vi "Dashboard Main.vi"() -> ()   [LabVIEW 2020]
uses:
  <vilib>/event_ctls.llb/eventvkey.ctl
  52f2dcef-b32f-41dc-9262-467f65fbdc6c.vi
  68ab9017-3ada-4b2c-b8c3-c0fcfab6ce46.vi
  <vilib>/Rock Robotics/Network Tables/NT Write Boolean.vi
  <vilib>/Rock Robotics/WPI/Dashboard/WPI_DashboardLogging Global.vi
  <vilib>/Analysis/NI_AALBase.lvlib
  <vilib>/Rock Robotics/Network Tables/NT Write Numeric Array.vi
panel:
  out "NT Connection":bool
  in  "Camera Settings Right":T1={"Frame Rate"=30, "Compression"=30, "Size"=1, "DB Camera Config"=FALSE} {"Frame Rate" scale=1.0..30.0; "Compression" scale=100.0..-1.0; "Size" items=["640x480", "320x240", "160x120"]}
  in  "Camera Name Right":string(combo)="No Camera Selection"
  out "Camera Perf":string
  in  "TCP":refnum<k5>
  in  "Rec Mode":enum32{"Stop", "Record", "Playback"}(radio)
  out "Robot IP":string
  out "Image Message":string="Timeout in Camera Communications"
  in  "Dashboard Tab":T2(tab)
  in  "Reset Climb":bool
  in  "Robot Selector":u16(ring) items=["2468", "2687"]
  out "Climb State":u16(ring) items=["Flip Hooks", "Rest Bar", "Tilt Back", "Tilt to Bar", "Grab Bar", "Pull Up"]
  out "Current Bar":u16(ring) items=["Ground", "Mid", "High", "Traverse"]
  in  "Calibrate (Reset Pods)":bool
  in  "Manual Paths":string[](array[string])
  in  "Ramping On?":bool
  in  "Max Rotation":dbl=540.0
  in  "Max Translation":dbl=15.0
  in  "Deadband":dbl=0.02
  out "Top Flywheel Voltage":dbl
  out "Auto Picture":picture
  in  "Auto Calibrate On?":bool=TRUE
  in  "Reset Hood":bool
  out "Main Flywheel RPM":dbl
  out "Hood Position":dbl
  in  "Auto Selector":T3(ring)
  out "IMU":dbl(knob) scale=-180.0..180.0
  out "Pivot Position":dbl
  out "Extension Position":dbl
  in  "Select Auto":string(combo)="Select Autonomous ..."
  out "Mode":T4(ring)=enum."Auto Disabled"
  out "Right Camera Perf":cluster{"Bandwidth (Mbps)":dbl, "FPS":dbl}
  in  "CheckList":i32(listbox)
  out "Climb State":u16(ring) items=["Flip Hooks", "Rest Bar", "Tilt Back", "Tilt to Bar", "Grab Bar", "Pull Up"]
  out "Current Shot":u16(ring) items=["Off", "Tarmac/Wall", "Protected"]
  out "Field Centric On?":bool
  out "Auto Align?":bool
  out "Background 2":bool
  out "Camera Image Right":T5(plugin-control)
  out "Tree":string(tree)
  out "Background":bool
  # "HW"
  # "IMU"
  # "Climb"
  # "Setup"
  # "Swerve"
  # "Shooter"
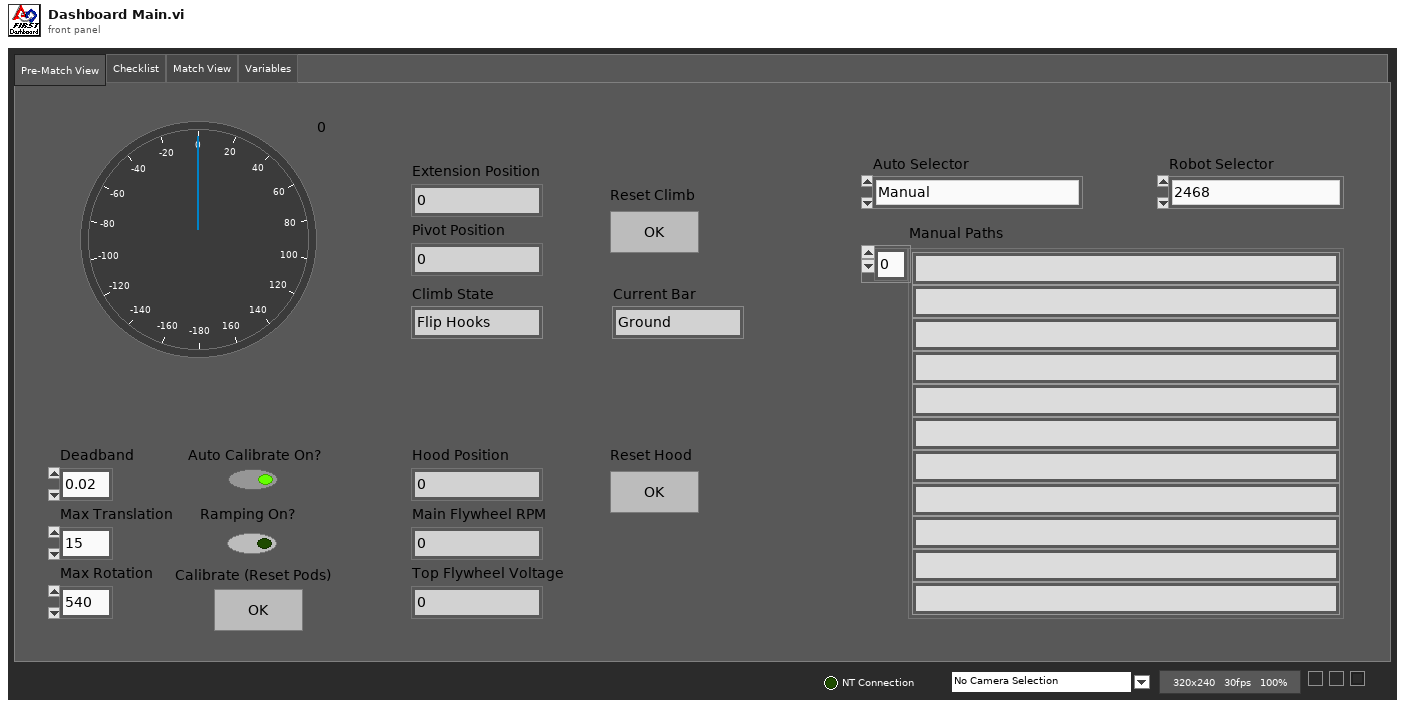
[diagram p1: front panel]
types:
  T1 = cluster{"Frame Rate":i32, "Compression":i32, "Size":u16, "DB Camera Config":bool}
  T2 = enum32{"Pre-Match View", "Checklist", "Match View", "Variables"}
  T3 = enum16{"Manual", "2 Ball Right", "5 Ball", "4 Ball Left", "4 Ball Right", "3 Ball", "2 Ball Left", "1 Ball"}
  T4 = enum8{"Tele-Op Disabled", "Tele-Op Enabled", "Auto Disabled", "Auto Enabled", "Test Disabled", "Test Enabled", "Disconnected", "No Code", "E-Stop"}
  T5 = typedef "IMAQ Image.ctl" = refnum<image>
  T6 = cluster{"Save Path":path, "Interval (s)":dbl, "Keep":i32}
  T7 = typedef "Image Type" = u32
  T8 = cluster{"IDs":cluster{"RPC field ID":u16, "Unique ID":u16}, "String":string}
  T9 = cluster{"Dashboard Tab":refnum<vi>, "Background":refnum<vi>, "Rec Mode":refnum<vi>, "Tree":refnum<vi>, "Camera Perf":refnum<vi>, "Camera Settings Right":refnum<vi>, "Camera Name Right":refnum<vi>, "Camera Image Right":refnum<vi>}
  T10 = cluster{"Global Rectangle":i32[], "Contours":cluster{"Contour Type":u32, "ROI Type":u32, "Points":i32[]}[]}
  T11 = cluster{"Camera Name Right":string, string, "Saved DB Images Info":cluster{"Save Path":path, "Interval (s)":dbl, "Keep":i32}}
  T12 = cluster{"Error Strings":string, "Disable Counts":cluster{u16, u16}, "Rail Faults":cluster{u16, u16, u16}, "Robot IP":string, "DB Mode":u8, "Event Info":cluster{"Name":string, "Type":u8, "Number":u16, "Replay":u8}}
  T13 = cluster{"Storage":cluster{"Disk Free":u64, "RAM Block":u32, "RAM free":u32}, "CPU Utilization":cluster{"CPU % ISR":sgl, "CPU % Time Crit":sgl, "CPU % Timed Str":sgl, "CPU % High":sgl, "CPU % Above":sgl, "CPU % Normal":sgl, "CPU % Low":sgl}, "CAN":cluster{"% Bus Utilization":sgl, "Bus Off Cnt":u32, "TX_FIFO Full Cnt":u32, "Receive Error Cnt":u8, "Transmit Error Cnt":u8}, "HID":cluster{"HID Outputs":u32, "Rumble Low":u16, "Rumble High":u16}[]}
  T14 = cluster{"Status bits":cluster{"Test Mode":bool, "Autonomous":bool, "Enabled":bool, "Code Start":bool, "Brownout":bool, "Reserved 2":bool, "Reserved 3":bool, "E-Stop":bool}, "Code Trace":cluster{"Disabled":bool, "TeleOp":bool, "Auto":bool, "Test":bool}, "Controller Type":enum16{"unknown", "cRIO", "roboRio"}, "Code?":enum16{"unknown", "noCode", "code"}, "Battery V":dbl}
  T15 = cluster{"Control Bits":cluster{"TestMode":bool, "Autonomous":bool, "Enabled":bool, "FMS Present":bool, bool, bool, bool, "E-Stop":bool}, "Team Station ":u8, "Countdown":sgl, "Joystick Values":cluster{"Axes":dbl[], "Buttons":bool[], "POVs":i16[]}[]}
  T16 = typedef "imagedata.ctl" = cluster{"image type":i32, "image depth":i32, "image":u8[], "mask":u8[], "colors":u32[], "Rectangle":cluster{"left":i16, "top":i16, "right":i16, "bottom":i16}}
  T17 = cluster{"Operation":enum16{"Update", "Clear"}, "Color Box":u32}[]
  T18 = typedef "eventvkey.ctl" = enum16{"ASCII", "Enter", "Return", "Shift", "Ctrl", "Alt", "Cmd", "Opt", "Caps", "NumLock", "Clear", "Break", "Up", "Down", "Left", "Right", "Insert", "Delete", "Home", "End", "PageUp", "PageDown", "Escape", "Help", "Pause", "ScrollLock", "F1", "F2", "F3", "F4", "F5", "F6", "F7", "F8", "F9", "F10", "F11", "F12", "F13", "F14", "F15", "F16", "F17", "F18", "F19", "F20", "F21", "F22", "F23", "F24", "Play", "VolumeUp", "VolumeDown", "Mute", "Two Byte Char"}
  T19 = cluster{"Image Size":bool, "Image Type":bool, "Pixel Value":bool, "ROI Information":bool, "Zoom Factor":bool}
  T20 = cluster{"Shift":bool, "Ctrl":bool, "Alt":bool, "Cmd":bool, "Opt":bool}
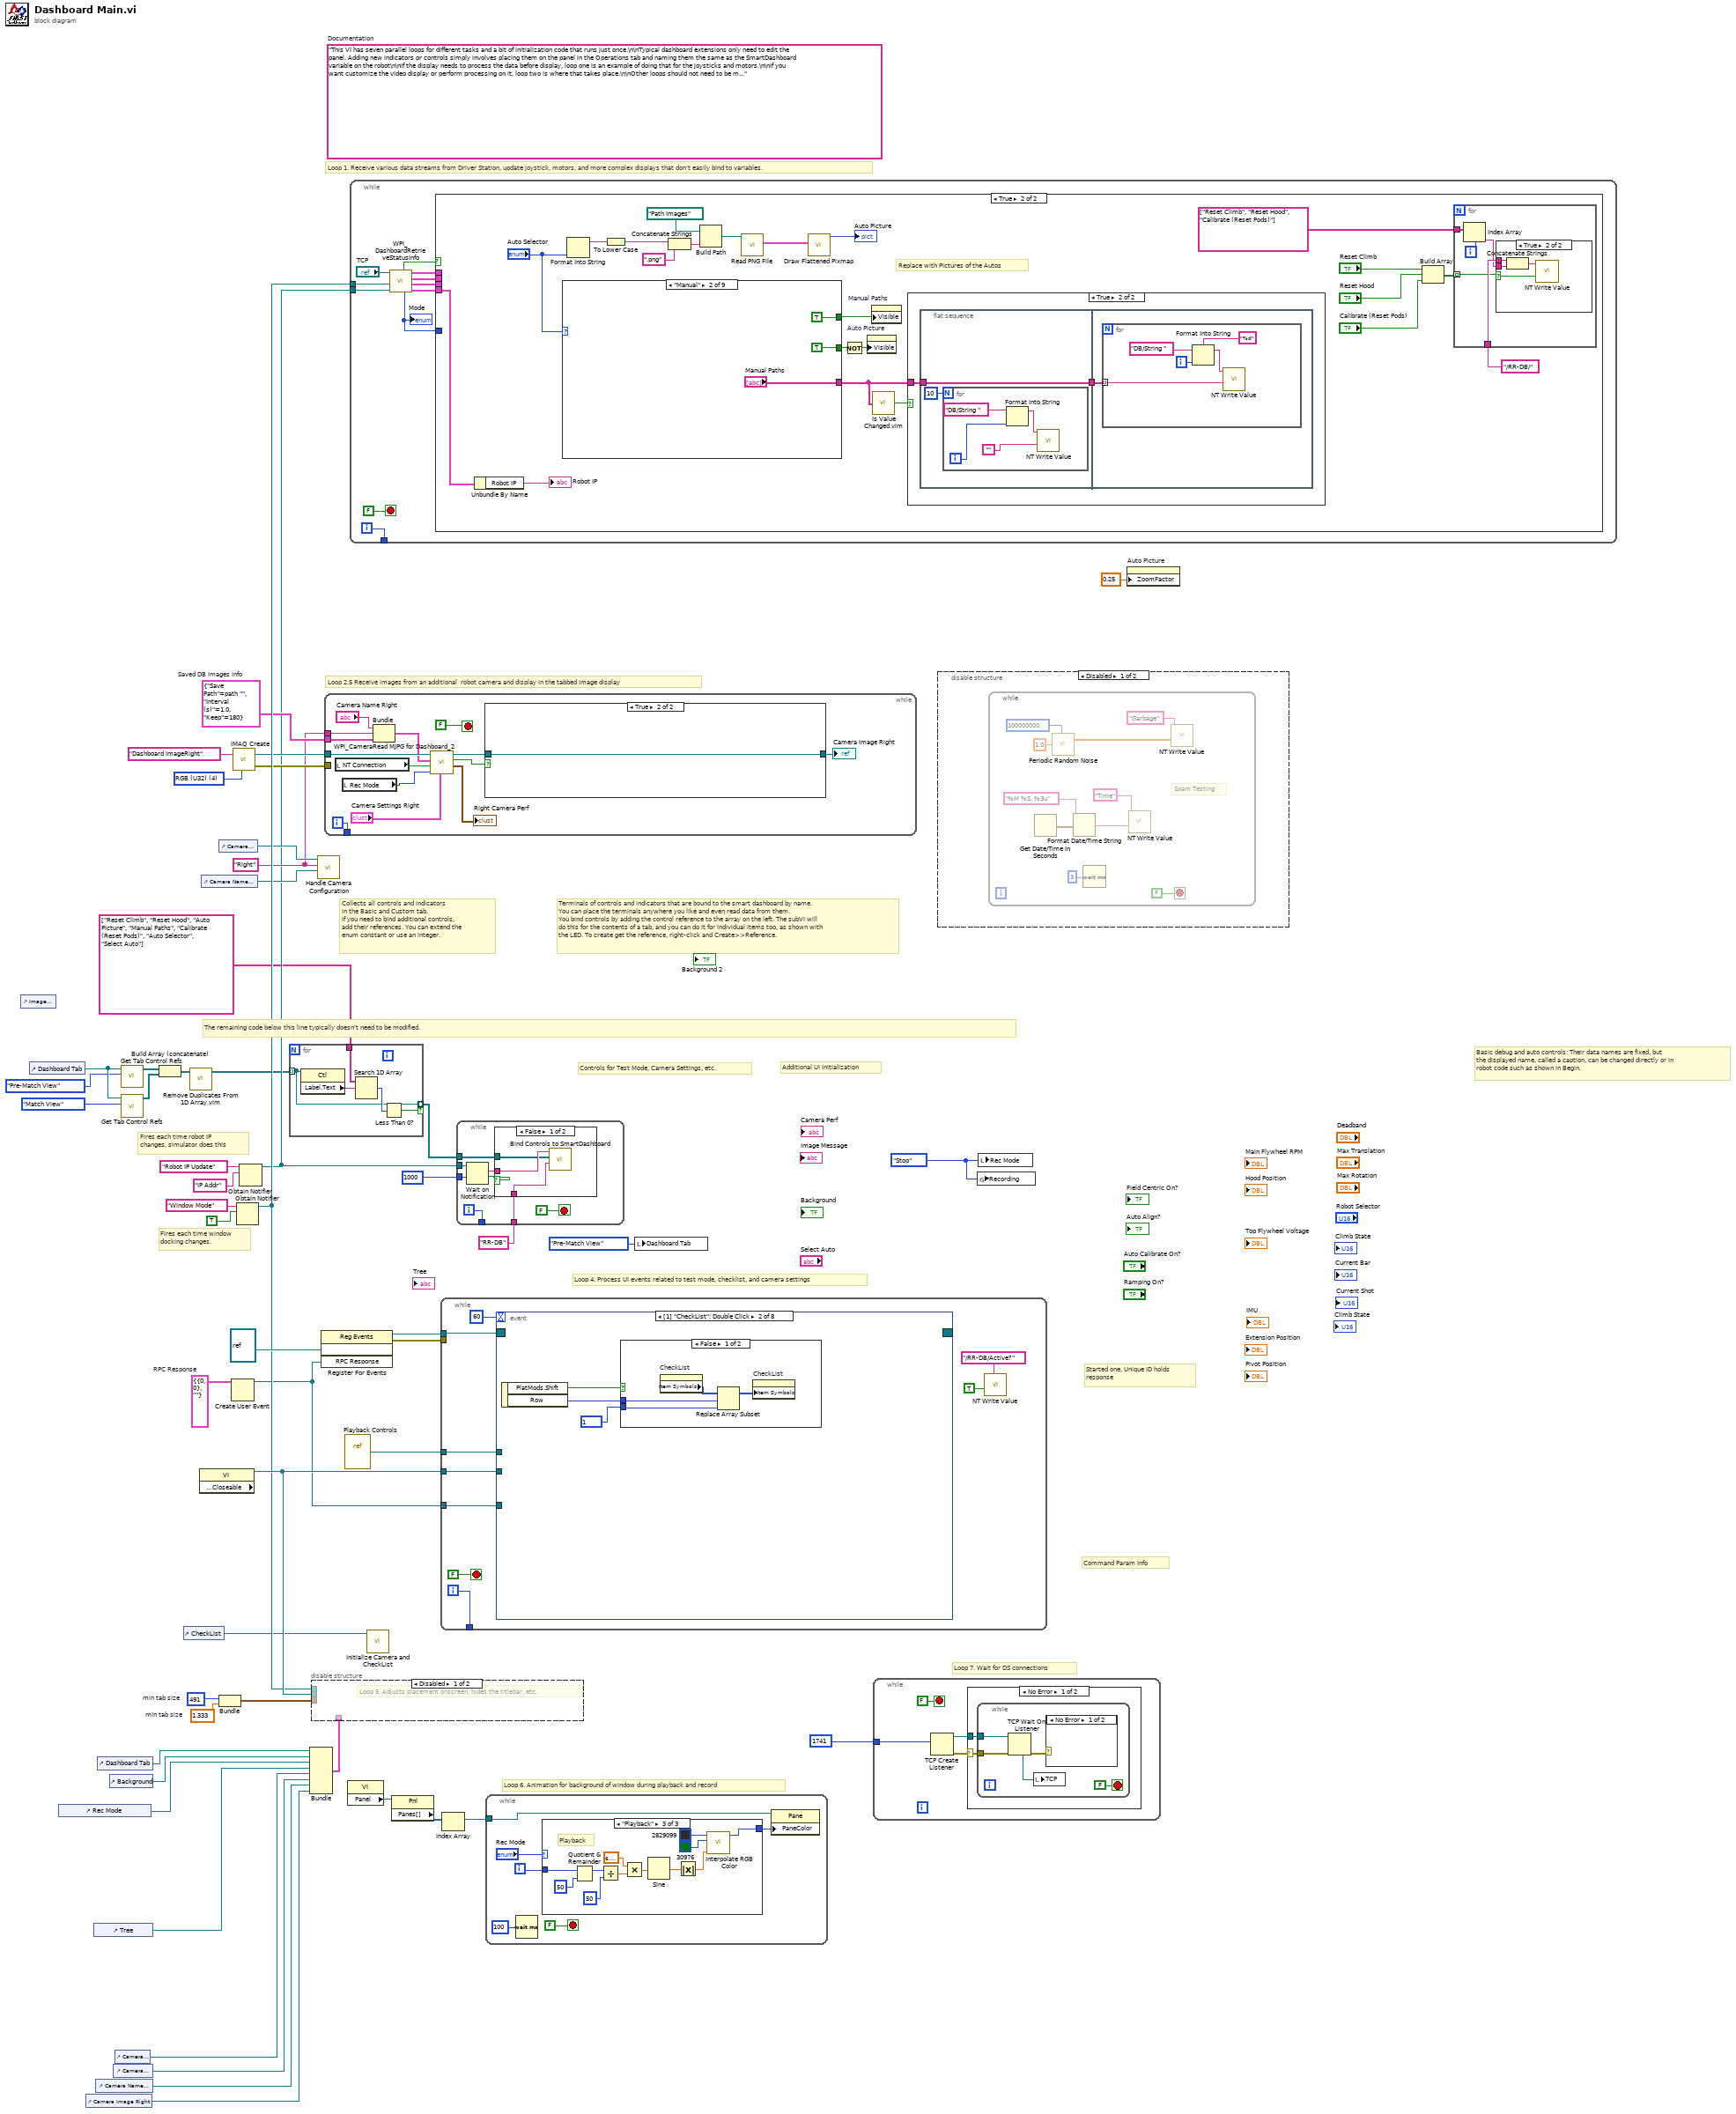
[diagram p0: block diagram]
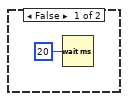
[diagram p3: hidden frame]
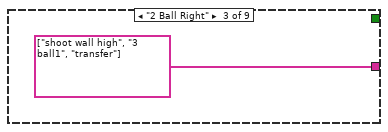
[diagram p7: hidden frame]
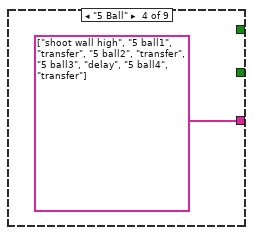
[diagram p8: hidden frame]
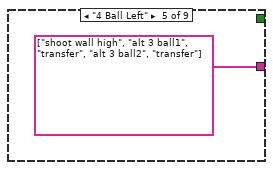
[diagram p9: hidden frame]
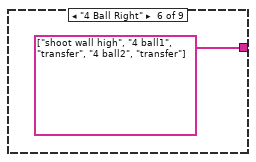
[diagram p10: hidden frame]
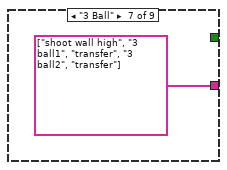
[diagram p11: hidden frame]
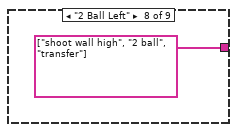
[diagram p12: hidden frame]
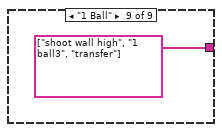
[diagram p13: hidden frame]
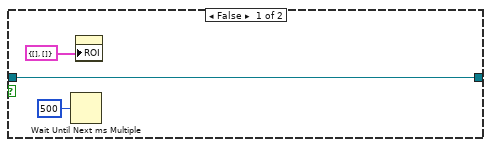
[diagram p16: hidden frame]
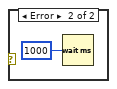
[diagram p17: hidden frame]
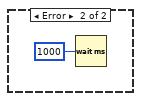
[diagram p18: hidden frame]
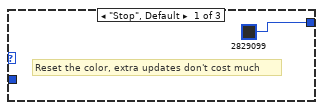
[diagram p19: hidden frame]
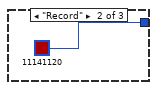
[diagram p20: hidden frame]
diagram:
  w18 = T6 {"Save Path"=path "", "Interval (s)"=1.0, "Keep"=180}  # Saved DB Images Info
  w17 = "Right"
  w26 = T7 4 items=["Grayscale (U8)", "Grayscale (I16)", "Grayscale (SGL)", "Complex (CSG)", "RGB (U32)", "HSL (U32)", "RGB (U64)"] ("Image Type")
  w30 = T8 {"IDs"={"RPC field ID"=0, "Unique ID"=0}, "String"=""}  # RPC Response
  w38 = 491  # min tab size
  w37 = 1.333  # min tab size
  w41 = enum32{"Stop", "Record", "Playback"}."Stop" ("Rec Mode")
  (unwired) "This VI has seven parallel loops for different tasks and a bit of initialization code that runs just once.\n\nTypical dashboard extensions only need to edit the panel. Adding new indicators or controls simply involves placing them on the panel in the Operations tab and naming them the same as the SmartDashboard variable on the robot\n\nIf the display needs to process the data before display, loop one is an example of doing that for the joysticks and motors.\n\nIf you want customize the video display or perform processing on it, loop two is where that takes place.\n\nOther loops should not need to be modified. They are pretty standard, and document the task they perform."  # Documentation
  # "Loop 2.5 Receive images from an additional  robot camera and display in the tabbed image display"
  # "Command Param Info"
  # "Started one, Unique ID holds\nresponse"
  # "Loop 7. Wait for DS connections"
  # "Basic debug and auto controls: Their data names are fixed, but\nthe displayed name, called a caption, can be changed directly or in\nrobot code such as shown in Begin."
  # "Controls for Test Mode, Camera Settings, etc."
  # "Additional UI Initialization"
  # "Loop 6. Animation for background of window during playback and record"
  # "Fires each time robot IP\nchanges, simulator does this"
  # "Fires each time window\ndocking changes."
  # "Collects all controls and indicators\nin the Basic and Custom tab.\nIf you need to bind additional controls,\nadd their references. You can extend the\nenum constant or use an integer."
  # "The remaining code below this line typically doesn't need to be modified."
  # "Loop 4. Process UI events related to test mode, checklist, and camera settings"
  # "Terminals of controls and indicators that are bound to the smart dashboard by name.\nYou can place the terminals anywhere you like and even read data from them.\nYou bind controls by adding the control reference to the array on the left. The subVI will\ndo this for the contents of a tab, and you can do it for individual items too, as shown with\nthe LED. To create get the reference, right-click and Create>>Reference."
  # "Loop 1. Receive various data streams from Driver Station, update joystick, motors, and more complex displays that don't easily bind to variables."
  n1 = control-ref of="Image Message"() -> ()  [unwired: 1 out]
  n2 = control-ref of="Dashboard Tab"() -> (w11:refnum<vi>)
  n3 = control-ref of="Rec Mode"() -> (w33:refnum<vi>)
  n4 = control-ref of="Camera Image Right"() -> (w19:refnum<vi>)
  n5 = control-ref of="Tree"() -> (w16:refnum<vi>)
  n6 = control-ref of="Camera Name Right"() -> (w20:refnum<vi>)
  n7 = control-ref of="Dashboard Tab"() -> (w39:refnum<vi>)
  n8 = control-ref of="Background"() -> (w35:refnum<vi>)
  n9 = control-ref of="Camera Settings Right"() -> (w21:refnum<vi>)
  n10 = control-ref of="Camera Perf"() -> (w28:refnum<vi>)
  n11 = call <vilib>:"Get Tab Control Refs.vi"("Page Index"=T2."Pre-Match View" ("Dashboard Tab"), "TabControl in"=w11) -> ("ControlsOnPage"=w10:refnum<vi>[])  [unwired: 9 in]
  n12 = call <vilib>:"Get Tab Control Refs.vi"("Page Index"=T2."Match View" ("Dashboard Tab"), "TabControl in"=w11) -> ("ControlsOnPage"=w9:refnum<vi>[])  [unwired: 9 in]
  n13 = Build Array (concatenate)(w10, w9) -> (w8:refnum<vi>[])
  n14 = control-ref of="CheckList"() -> (w12:refnum<vi>)
  n15 = call "Remove Duplicates From 1D Array.vim"("array"=w8) -> ("array with duplicates removed"=w5:refnum<vi>[])  [unwired: 10 in]
  n16 = property class="VI" props=["Front Panel.Closeable"]() -> (reference out=w40:refnum<vi>)  [unwired: 2 in, 2 out]
  n17 = control-ref of="Camera Name Right"() -> (w22:refnum<vi>)
  n18 = control-ref of="Camera Settings Right"() -> (w23:refnum<vi>)
  n19 = Bundle("min tab size"=w38, "min tab size"=w37) -> (w36:cluster{"min tab size":i32, "min tab size":dbl})  [unwired: 1 in]
  n20 = Create User Event(user event datatype=w30) -> (user event=w29:refnum<user-event>)  [unwired: 1 in, 1 out]
  n21 = call "IMAQ Create"("Image Name"="Dashboard ImageRight", "Image Type"=w26) -> ("New Image"=w25:T5, "error out"=w24:errorcluster)  [unwired: 2 in, 1 out]
  n22 = Obtain Notifier(name (unnamed)="Window Mode", notification data type=TRUE) -> (notifier out=w32:refnum<notifier>)  [unwired: 2 in, 2 out]
  n23 = Obtain Notifier(name (unnamed)="Robot IP Update", notification data type="IP Addr" ("name (unnamed)")) -> (notifier out=w14:refnum<notifier>)  [unwired: 2 in, 2 out]
  n24 = for {
    tunnel: string[] ["Reset Climb", "Reset Hood", "Auto Picture", "Manual Paths", "Calibrate (Reset Pods)", "Auto Selector", "Select Auto"] -> [w57]
    tunnel: w5 -> [w54] mode=indexing
    tunnel: [w54] -> w4 mode=indexing if=w53
    n25 = property class="Ctl"(reference=w54) -> ("Label.Text"=w56:string)  [unwired: 1 in, 2 out]
    n26 = Search 1D Array(1D array=w57, element=w56) -> (index of element=w55:i32)  [unwired: 1 in]
    n27 = Less Than 0?(x=w55) -> (x < 0?=w53:bool)
  }
  n28 = Bundle("Dashboard Tab"=w39, "Background"=w35, "Rec Mode"=w33, "Tree"=w16, "Camera Perf"=w28, "Camera Settings Right"=w21, "Camera Name Right"=w20, "Camera Image Right"=w19) -> (w34:T9)  [unwired: 1 in]
  n29 = disable-structure shown="Disabled" {
    disable-tunnel: w40 -> [_ _]
    disable-tunnel: w36 -> [_ _]
    disable-tunnel: w34 -> [_ _]
    disable-tunnel: w32 -> [_ _]
    frame Disabled {
      # "Loop 5. Adjusts placement onscreen, hides the titlebar, etc."
    }
    frame Enabled {
    }
  }
  n30 = call "Handle Camera Configuration.vi"("CameraNameRef"=w22, "Display Name"=w17, "ClusterRef"=w23) -> ()  [unwired: 9 in]
  n31 = register-events(refnum<vi> refnum, w29) -> (reference out=w44:refnum<event-registration>, error out=w43:errorcluster)  [unwired: 2 in]
  n32 = while {
    tunnel: w25 -> [w71]
    tunnel: w24 -> [_]
    tunnel: [w66] -> _
    tunnel: w18 -> [w62]
    tunnel: w17 -> [w59]
    i -> [w66]
    stop <- FALSE stop-if-true
    n33 = local read "NT Connection"() -> (w63:bool)
    n34 = local read "Rec Mode"() -> (w70:enum32{"Stop", "Record", "Playback"})
    n35 = Bundle("Camera Name Right"="Camera Name Right", w59, "Saved DB Images Info"=w62) -> (w61:T11)  [unwired: 1 in]
    n36 = call <vilib>:"WPI_CameraRead MJPG for Dashboard_2.vi"("Camera Settings"="Camera Settings Right", "Rec Mode"=w70, "NT Connection"=w63, "Capture Info"=w61, "Image in"=w71) -> ("perf info"=→"Right Camera Perf":cluster{"Bandwidth (Mbps)":dbl, "fps":dbl}, "Active"=w65:bool, "Image\\ out"=w68:T5)  [unwired: 4 in]
    n37 = case shown="True" w65 {
      tunnel: w68 -> [w73 w75]
      tunnel: [w73 w75] -> w64
      frame False {
        n38 = Wait Until Next ms Multiple(millisecond multiple=u32 500) -> ()  [unwired: 1 out]
        n39 = property on="Camera Image Right" class="ImageControl"("ROI"=T10 {"Global Rectangle"=[], "Contours"=[]}) -> ()  [unwired: 2 in, 2 out]
      }
      frame True {
      }
    }
    "Camera Image Right" <- w64
  }
  n40 = vi-ref "Playback Controls.vi"() -> (w45:refnum<vi>)
  n41 = property class="VI"() -> ("Panel"=w47:refnum<vi>)  [unwired: 2 in, 2 out]
  n42 = while {
    tunnel: [w85] -> _
    tunnel: w14 -> [w79]
    tunnel: w32 -> [w76]
    i -> [w85]
    stop <- FALSE stop-if-true
    n43 = call <vilib>:"WPI_DashboardRetrieveStatusInfo.vi"("Binding Refnum"=w79, "Window Mode Notifier"=w76, "TCP Cnx"="TCP") -> ("Power and Errors"=w80:T12, "Robot Metrics"=w83:T13, "Status Info"=w84:T14, "Control Info"=w81:T15, "Robot Mode"=w78:T4, "Process?"=w82:bool)  [unwired: 3 in]
    "Mode" <- w78
    n44 = case shown="True" w82 {
      tunnel: w84 -> [_ _]
      tunnel: w83 -> [_ _]
      tunnel: w81 -> [_ _]
      tunnel: w80 -> [_ w109]
      tunnel: w78 -> [_ _]
      frame False {
        n45 = Wait (ms)(milliseconds to wait=u32 20) -> ()  [unwired: 1 out]
      }
      frame True {
        # "Replace with Pictures of the Autos"
        n46 = Unbundle By Name(w109) -> ("Robot IP"=→"Robot IP":string)
        n47 = case shown="\"Manual\"" "Auto Selector" {
          tunnel: [_ "Manual Paths" string[] ["shoot wall high", "3 ball1", "transfer"] string[] ["shoot wall high", "5 ball1", "transfer", "5 ball2", "transfer", "5 ball3", "delay", "5 ball4", "transfer"] string[] ["shoot wall high", "alt 3 ball1", "transfer", "alt 3 ball2", "transfer"] string[] ["shoot wall high", "4 ball1", "transfer", "4 ball2", "transfer"] string[] ["shoot wall high", "3 ball1", "transfer", "3 ball2", "transfer"] string[] ["shoot wall high", "2 ball", "transfer"] string[] ["shoot wall high", "1 ball3", "transfer"]] -> w107
          tunnel: [_ TRUE ("Visible") _ _ _ _ _ _ _] -> w98
          tunnel: [_ TRUE ("Visible") _ _ _ _ _ _ _] -> w96
          frame Default {
          }
          frame "Manual" {
          }
          frame "2 Ball Right" {
          }
          frame "5 Ball" {
          }
          frame "4 Ball Left" {
          }
          frame "4 Ball Right" {
          }
          frame "3 Ball" {
          }
          frame "2 Ball Left" {
          }
          frame "1 Ball" {
          }
        }
        n48 = Format Into String("Auto Selector") -> (resulting string=w105:string)  [unwired: 3 in, 1 out]
        n49 = To Lower Case(string=w105) -> (all lower case string=w104:string)
        n50 = Concatenate Strings(w104, ".png" ("string")) -> (w103:string)
        n51 = Build Path(base path=path "Path Images", name or relative path=w103) -> (appended path=w102:path)
        n52 = call <vilib>:"Read PNG File.vi"("path to PNG file"=w102) -> ("image data"=w101:T16)  [unwired: 8 in, 2 out]
        n53 = call <vilib>:"Draw Flattened Pixmap.vi"("image data"=w101) -> ("new picture"=→"Auto Picture":picture)  [unwired: 8 in]
        n54 = Not(x=w98) -> (.not. x?=w97:bool)
        n55 = property on="Auto Picture" class="Pict"("Visible"=w97) -> ()  [unwired: 2 in, 2 out]
        n56 = property on="Manual Paths" class="Arr (strict)"("Visible"=w96) -> ()  [unwired: 2 in, 2 out]
        n57 = call "Is Value Changed.vim"("value"=w107) -> ("changed or first call?"=w106:bool)
        n58 = case shown="True" w106 {
          tunnel: w107 -> [_ w120]
          frame False {
          }
          frame True {
            n59 = flat-sequence {
              tunnel: w120 -> [w122]
              tunnel: [w122] -> w119
              tunnel: w119 -> [w127]
              frame #0 {
                n60 = for {
                  N: 10 -> [_]
                  i -> [w125]
                  n61 = Format Into String(initial string="DB/String ", w125) -> (resulting string=w124:string)  [unwired: 2 in, 1 out]
                  n62 = call-poly <vilib>:"NT Write Value.vi"("String"="", "Name"=w124) -> ()  [unwired: 9 in, 1 out]
                }
              }
              frame #1 {
                n63 = for {
                  tunnel: w127 -> [w129] mode=indexing
                  i -> [w132]
                  n64 = Format Into String(format string="%d", initial string="DB/String ", w132) -> (resulting string=w130:string)  [unwired: 1 in, 1 out]
                  n65 = call-poly <vilib>:"NT Write Value.vi"("String"=w129, "Name"=w130) -> ()  [unwired: 9 in, 1 out]
                }
              }
            }
          }
        }
        n66 = Build Array("Reset Climb", "Reset Hood", "Calibrate (Reset Pods)") -> (w91:bool[])
        n67 = for {
          tunnel: "/RR-DB/" ("Name") -> [w114]
          tunnel: w91 -> [w110] mode=indexing
          tunnel: string[] ["Reset Climb", "Reset Hood", "Calibrate (Reset Pods)"] -> [w112]
          i -> [w113]
          n68 = Index Array(array=w112, index=w113) -> (element=w111:string)
          n69 = case shown="True" w110 {
            selector: w110 -> [_ w115]
            tunnel: w114 -> [_ w117]
            tunnel: w111 -> [_ w116]
            frame False {
            }
            frame True {
              n70 = Concatenate Strings(w117, w116) -> (w118:string)
              n71 = call-poly <vilib>:"NT Write Value.vi"("Boolean"=w115, "Name"=w118) -> ()  [unwired: 9 in, 1 out]
            }
          }
        }
      }
    }
  }
  n72 = call "Initialize Camera and CheckList.vi"("ListBox in"=w12) -> ()  [unwired: 11 in]
  n73 = property class="Pnl"(reference=w47) -> ("Panes[]"=w48:refnum<vi>[])  [unwired: 1 in, 2 out]
  n74 = while {
    tunnel: [w149] -> _
    tunnel: w45 -> [w148]
    tunnel: w44 -> [w147]
    tunnel: w43 -> [_]
    tunnel: w40 -> [w146]
    tunnel: w29 -> [w145]
    i -> [w149]
    stop <- FALSE stop-if-true
    n75 = event shown="[1] \"CheckList\": Double Click" {
      selector: w147 -> [_ _ _ _ _ _ _ _]
      dyn-events: [_ _ _ _ _ w195 _ _] -> _
      timeout: u32 60 ("milliseconds to wait") -> [_ _ _ _ _ _ _ _]
      tunnel: w148 -> [_ _ _ _ _ w197 w212 _]
      tunnel: w146 -> [_ _ _ _ _ w193 _ _]
      tunnel: w145 -> [_ _ _ _ _ w191 _ _]
      event Timeout {
        n76 = event-data() -> ()  [unwired: 1 in, 1 out]
        n77 = local read "Mode"() -> (w154:T4)
        n78 = case shown="\"Variables\"" "Dashboard Tab" {
          tunnel: "TestMode/Automatic/" ("Name Pattern") -> [_ _]
          tunnel: T17 [{"Operation"=enum."Clear", "Color Box"=14013909}, {"Operation"=enum."Clear", "Color Box"=14013909}, {"Operation"=enum."Clear", "Color Box"=14013909}, {"Operation"=enum."Clear", "Color Box"=14013909}, {"Operation"=enum."Update", "Color Box"=14013909}, {"Operation"=enum."Update", "Color Box"=16777215}, {"Operation"=enum."Clear", "Color Box"=14013909}, {"Operation"=enum."Clear", "Color Box"=14013909}, {"Operation"=enum."Clear", "Color Box"=14013909}] -> [_ _]
          tunnel: w154 -> [_ _]
          tunnel: u32[] [15790320, 15790320, 15790320, 15790320, 16777215, 16777215, 15790320, 15790320, 15790320] -> [_ _]
          frame Default {
          }
          frame "Variables" {
            w160 = string[] ["CameraPublisher", "Usage", "DB"]  # Items to initially close
            n79 = First Call?() -> (First Call?: T/F=w161:bool)
            n80 = control-ref of="Tree"() -> (w162:refnum<vi>)
            n81 = Select(t=w160, s=w161, f=string[] []) -> (s? t:f=w158:string[])
            n82 = call <vilib>:"NT Read and Format Entries as Tree.vi"("Tags to  Close"=w158, "Tree Refnum"=w162) -> ()  [unwired: 8 in, 2 out]
          }
        }
        n83 = call <vilib>:"Connextion Info.vi"() -> ("Connected"=→"NT Connection":bool)  [unwired: 10 in, 1 out]
      }
      event "CheckList": Double Click {
        n84 = event-data() -> ("PlatMods.Shift"=w164:bool, "Row"=w163:i32)  [unwired: 1 in]
        n85 = case shown="False" w164 {
          tunnel: w163 -> [w167 _]
          tunnel: 1 -> [w166 _]
          frame False {
            n86 = property on="CheckList" class="LstBox (strict)"() -> ("Item Symbols"=w168:i32[])  [unwired: 2 in, 2 out]
            n87 = Replace Array Subset(array=w168, new element=w166, index=w167) -> (w169:i32[])
            n88 = property on="CheckList" class="LstBox (strict)"("Item Symbols"=w169) -> ()  [unwired: 2 in, 2 out]
          }
          frame True {
            w171 = 0 ("Top Row")
            n89 = property on="CheckList" class="LstBox (strict)"() -> ("Number of Rows"=w172:u32)  [unwired: 2 in, 2 out]
            n90 = Initialize Array(0, w172) -> (w170:i32[])
            n91 = property on="CheckList" class="LstBox (strict)"("Top Row"=w171, "Value"=w171, "Item Symbols"=w170) -> ()  [unwired: 2 in, 2 out]
          }
        }
      }
      event "CheckList": Key Down {
        n92 = event-data() -> ("VKey"=w174:T18)  [unwired: 1 in]
        n93 = case shown="\"Left\", \"Right\"" w174 {
          selector: w174 -> [w183 _]
          tunnel: eventvkey."Left" ("VKey") -> [w181 _]
          frame "Left", "Right" {
            n94 = Equal?(x=w181, y=w183) -> (x = y?=w182:bool)
            n95 = Select(t=0, s=w182, f=1) -> (s? t:f=w184:i32)
            n96 = property on="CheckList" class="LstBox (strict)"() -> ("Item Symbols"=w177:i32[])  [unwired: 2 in, 2 out]
            n97 = Replace Array Subset(array=w177, new element=w184, index="CheckList") -> (w176:i32[])
            n98 = property on="CheckList" class="LstBox (strict)"("Item Symbols"=w176) -> ()  [unwired: 2 in, 2 out]
          }
          frame Default {
          }
        }
      }
      event "Select Auto": Mouse Enter {
        # "Populate the combo box with the list of autonomous options"
        n99 = event-data() -> ()  [unwired: 1 in, 1 out]
        n100 = call <vilib>:"NT Read String Array.vi"("Name"="Auto List") -> ("String Array"=w185:string[])  [unwired: 9 in, 1 out]
        n101 = property on="Select Auto" class="CmbBox"("Strings[]"=w185) -> ()  [unwired: 2 in, 2 out]
      }
      event "Select Auto": Value Change {
        # "User modified the Auto Selection. Write to NT variable so robot knows."
        n102 = event-data() -> ("NewVal"=w187:string)  [unwired: 1 in]
        n103 = call <vilib>:"NT Write String.vi"("String"=w187, "Name"="Auto Selector") -> ()  [unwired: 9 in, 1 out]
      }
      event "Rec Mode": Value Change {
        # "Update globals for recording mode and path to read log from.\nClear when logging and let NetworkTables set path for vision to\nuse."
        n104 = event-data() -> ("NewVal"=w198:enum32{"Stop", "Record", "Playback"})  [unwired: 1 in]
        n105 = global write "WPI_DashboardLogging Global.vi" "Logging Filename"(path "") -> ()
        n106 = global write "WPI_DashboardLogging Global.vi" "Recording"(w198) -> ()
        n107 = case shown="\"Playback\"" w198 {
          tunnel: w197 -> [_ w200 w209]
          tunnel: [_ _ w208] -> w195
          tunnel: [_ _ w207] -> _
          tunnel: w193 -> [_ _ w205]
          tunnel: cluster{i32, i32} {-250, 170} -> [_ _ w204]
          tunnel: [_ _ T19 {"Image Size"=TRUE, "Image Type"=TRUE, "Pixel Value"=TRUE, "ROI Information"=TRUE, "Zoom Factor"=FALSE} ("Image Information Shown:All Elements")] -> w189
          tunnel: [_ _ TRUE ("Zoom Factor")] -> w190
          tunnel: w191 -> [_ _ w201]
          frame Default {
          }
          frame "Stop", "Record" {
            # "Place Window too"
            n108 = invoke class="VI" method="FP.Close"(reference=w200) -> (reference out=w199:refnum<vi>)  [unwired: 2 in, 2 out]
            n109 = invoke class="VI" method="Abort VI"(reference=w199) -> ()  [unwired: 2 in, 3 out]
          }
          frame "Playback" {
            n110 = call "Open Playback Panel.vi"("Offset"=w204, "DB VI Ref"=w205, "Playback in"=w209) -> ("Playback out"=w206:refnum<vi>)  [unwired: 8 in]
            n111 = register-events(w206, w201) -> (reference out=w208:refnum<event-registration>, error out=w207:errorcluster)  [unwired: 2 in]
          }
        }
        n112 = property on="Camera Image Right" class="ImageControl"("Image Information Shown"=w189, "Image Information Visible"=w190) -> ()  [unwired: 2 in, 2 out]
        n113 = call <vilib>:"WPI_DashboardNT Log FieldName Cache.vi"("Operation"=enum16{"Lookup/Add", "Index", "Clear"}."Clear") -> ()  [unwired: 8 in, 3 out]
      }
      event Panel Close {
        # "Abort playback window and ourself"
        n114 = event-data() -> ()  [unwired: 1 in, 4 out]
        n115 = invoke class="VI" method="FP.Close"(reference=w212) -> (reference out=w211:refnum<vi>)  [unwired: 2 in, 2 out]
        n116 = invoke class="VI" method="Abort VI"(reference=w211) -> (error out=w210:errorcluster)  [unwired: 2 in, 2 out]
        n117 = invoke class="VI" method="Abort VI"(error in=w210) -> ()  [unwired: 2 in, 3 out]
      }
      event "Tree": Double Click {
        n118 = event-data() -> ("PlatMods"=w218:T20, "Tag"=w215:string)  [unwired: 1 in]
        n119 = Unbundle(w218) -> ("Shift"=w217:bool)  [unwired: 4 out]
        n120 = String Subset(string=w215, length (rest)=1 ("length (rest)")) -> (substring=w214:string)  [unwired: 1 in]
        n121 = Not(x=w217) -> (.not. x?=w216:bool)
        n122 = case shown="\"/\"" w214 {
          tunnel: w215 -> [_ w220]
          tunnel: w216 -> [_ w219]
          frame Default {
          }
          frame "/" {
            n123 = call <vilib>:"NT Update Persistence.vi"("Persistence"=w219, "Name"=w220) -> ()  [unwired: 9 in, 1 out]
          }
        }
      }
    }
    n124 = call-poly <vilib>:"NT Write Value.vi"("Boolean"=TRUE, "Name"="/RR-DB/Active?") -> ()  [unwired: 9 in, 1 out]
  }
  n125 = Index Array(array=w48) -> (element=w46:refnum<vi>)  [unwired: 1 in]
  n126 = while {
    tunnel: w14 -> [w227]
    tunnel: [w225] -> _
    tunnel: u32 1000 ("milliseconds to wait") -> [w224]
    tunnel: w4 -> [w222]
    tunnel: "RR-DB" ("Path Prefix") -> [w221]
    i -> [w225]
    stop <- FALSE stop-if-true
    n127 = Wait on Notification(notifier=w227, timeout in ms (-1)=w224) -> (notification=w226:string, timed out?=w223:bool)  [unwired: 2 in, 2 out]
    n128 = case shown="False" w223 {
      tunnel: w226 -> [w231 _]
      tunnel: w222 -> [w230 _]
      tunnel: w221 -> [w229 _]
      frame False {
        n129 = call <vilib>:"Bind Controls to SmartDashboard.vi"("Path Prefix"=w229, "Bound Control Refs"=w230, "Server IP Address"=w231) -> ()  [unwired: 9 in]
      }
      frame True {
      }
    }
  }
  n130 = while {
    tunnel: w46 -> [w233]
    i -> [w236]
    stop <- FALSE stop-if-true
    n131 = Wait (ms)(milliseconds to wait=u32 100) -> ()  [unwired: 1 out]
    n132 = case shown="\"Playback\"" "Rec Mode" {
      tunnel: w236 -> [_ _ w251]
      tunnel: [u32 2829099 ("Base Color") u32 11141120 ("Target Color") w240] -> w232
      frame "Stop", Default {
        # "Reset the color, extra updates don't cost much"
      }
      frame "Record" {
      }
      frame "Playback" {
        # "Playback"
        n133 = Quotient & Remainder(x=w251, y=u32 50 ("milliseconds to wait")) -> (x-y*floor(x/y)=w247:u32)  [unwired: 1 out]
        n134 = Divide(x=w247, y=u32 50 ("milliseconds to wait")) -> (x/y=w244:dbl)
        n135 = Multiply(x=6.283185307179586, y=w244) -> (x*y=w249:dbl)
        n136 = Sine(x=w249) -> (sin(x)=w248:dbl)
        n137 = Absolute Value(x=w248) -> (abs(x)=w241:dbl)
        n138 = call "Interpolate RGB Color.vi"("Proportion"=w241, "Target Color"=u32 30976, "Base Color"=u32 2829099) -> ("Result Color"=w240:u32)  [unwired: 8 in]
      }
    }
    n139 = property class="Pane"(reference=w233, "PaneColor"=w232) -> ()  [unwired: 1 in, 2 out]
  }
  n140 = local write "Dashboard Tab"(T2."Pre-Match View" ("Dashboard Tab")) -> ()
  n141 = while {
    tunnel: u16 1741 ("timeout ms (25000)") -> [w253]
    stop <- FALSE stop-if-true
    n142 = TCP Create Listener(10:w253) -> (0:w252:errorcluster, 3:w254:refnum<k5>)  [unwired: 4 in, 1 out]
    n143 = case shown="No Error" w252 {
      selector: w252 -> [w256 _]
      tunnel: w254 -> [w257 _]
      frame No Error {
        n144 = while {
          tunnel: w257 -> [w260]
          tunnel: w256 -> [w259]
          stop <- FALSE stop-if-true
          n145 = TCP Wait On Listener(8:w259, 11:w260) -> (0:w261:errorcluster, 4:w262:refnum<k5>)  [unwired: 2 in, 3 out]
          n146 = local write "TCP"(w262) -> ()
          n147 = case shown="No Error" w261 {
            frame No Error {
            }
            frame Error {
              n148 = Wait (ms)(milliseconds to wait=u32 1000) -> ()  [unwired: 1 out]
            }
          }
        }
      }
      frame Error {
        n149 = Wait (ms)(milliseconds to wait=u32 1000) -> ()  [unwired: 1 out]
      }
    }
  }
  n150 = disable-structure shown="Disabled" {
    frame Disabled {
      n151 = while {
        stop <- FALSE stop-if-true
        # "Spam Testing"
        n152 = Get Date/Time In Seconds() -> (seconds since 1Jan1904=w271:timestamp)
        n153 = call <vilib>:"Periodic Random Noise.vi"("spectral amplitude"=1.0, "samples"=100000000) -> ("periodic random noise"=w266:dbl[])  [unwired: 1 in, 1 out]
        n154 = Format Date/Time String(time format string (%c)="%M %S, %3u", seconds (now)=w271) -> (date/time string=w270:string)  [unwired: 1 in]
        n155 = Wait (ms)(milliseconds to wait=u32 3) -> ()  [unwired: 1 out]
        n156 = call-poly <vilib>:"NT Write Value.vi"("String"=w270, "Name"="Time") -> ()  [unwired: 9 in, 1 out]
        n157 = call-poly <vilib>:"NT Write Value.vi"("Numeric Array"=w266, "Name"="Garbage") -> ()  [unwired: 9 in, 1 out]
      }
    }
    frame Enabled {
    }
  }
  n158 = global write "WPI_DashboardLogging Global.vi" "Recording"(w41) -> ()
  n159 = local write "Rec Mode"(w41) -> ()
  n160 = property on="Auto Picture" class="Pict"("ZoomFactor"=sgl 0.25 ("Zoom Factor")) -> ()  [unwired: 2 in, 2 out]
